vi "DisplayPosition.vi"(8 "error in":errorcluster, 10 "Current Position:":refnum<vi>, 11 "CmdLib In":refnum<k24>) -> (0 "error out":errorcluster, 3 "CmdLib Out":refnum<k24>)   [LabVIEW 2018]
uses:
  CmdLib.dll
  Global Variables.vi
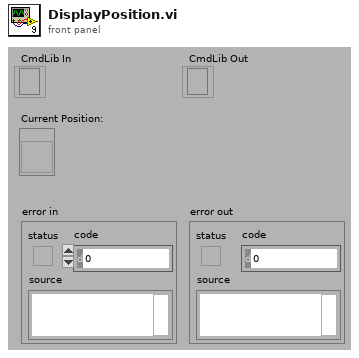
[diagram p1: front panel]
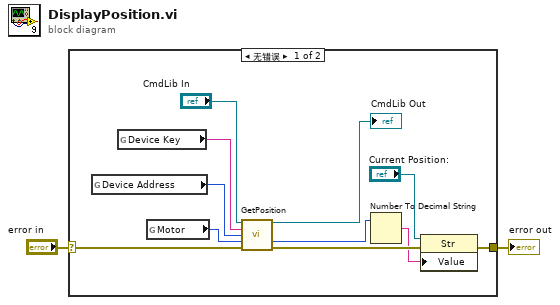
[diagram p0: block diagram]
diagram:
  n1 = case shown="无错误" "error in" {
    selector: "error in" -> [w6 w14]
    tunnel: [w12 w14] -> w2
    frame No Error {
      n2 = global read "Global Variables.vi" "Device Address"() -> (w3:i32)
      n3 = global read "Global Variables.vi" "Device Key"() -> (w5:string)
      n4 = global read "Global Variables.vi" "Motor"() -> (w4:i32)
      n5 = call "GetPosition.vi"("CmdLib In"="CmdLib In", "DeviceKey In"=w5, "Device Address In"=w3, "Motor"=w4, "error in (no error)"=w6) -> ("CmdLib Out"=→"CmdLib Out":refnum<k24>, "Position"=w10:i32, "error out"=w13:errorcluster)  [unwired: 6 in, 2 out]
      n6 = Number To Decimal String(number=w10) -> (decimal integer string=w9:string)  [unwired: 1 in]
      n7 = property class="Str"(reference="Current Position:", error in=w13, "Value"=w9) -> (error out=w12:errorcluster)  [unwired: 1 out]
    }
    frame Error {
    }
  }
  "error out" <- w2
